vi "Assert 1D Array wired to 1D Array Type.vi"   [LabVIEW 2017]
uses:
  e3e81a85-29a2-4e47-b418-2af2e786c2d5.vi
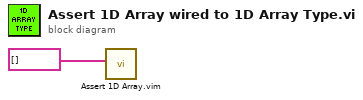
[diagram p0: block diagram]
diagram:
  n1 = call "Assert 1D Array.vim"("Array in"=string[] []) -> ()  [unwired: 10 in, 1 out]
